vi "Decode Response.vi"(6 "error in (no error)":errorcluster, 9 "output cluster in":T1) -> (0 "error out":errorcluster, 3 "output cluster out":T1)   [LabVIEW 2020]
uses:
  Data Cluster.ctl
  <vilib>/Utility/miscctls.llb/LVDateTimeRec.ctl
panel:
  out "NumSamples":u8
  out "Samples (new, old, older)":u8[](array[numeric]) format="%02x"
  out "Status":u8
  out "Offset":u8
  out "Range":u8
  out "Sample (new)":sgl
  out "Sample (old)":sgl
  out "Sample (older)":sgl
  out "Mo":sgl
  out "unsigned byte array":u8[](array[numeric])
  out "Mf":sgl
  # "Send Data:"
  # "Receive Data:"
  # "Send Data:"
  # "Receive Data:"
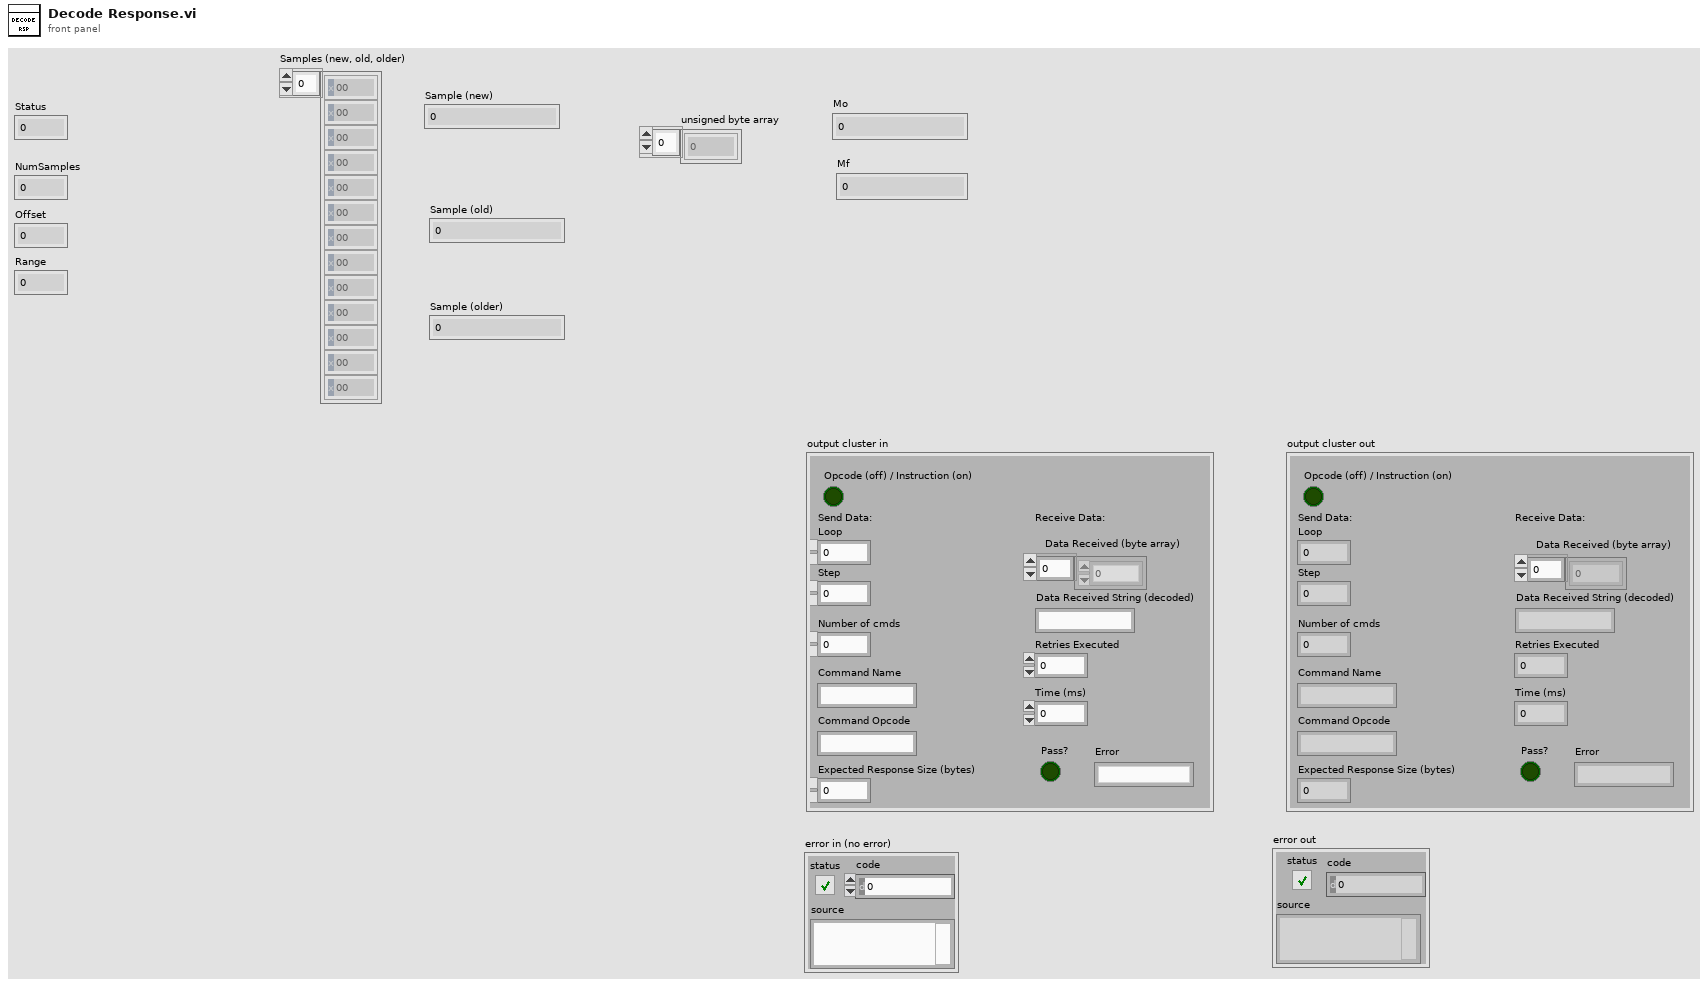
[diagram p1: front panel]
types:
  T1 = typedef "Data Cluster.ctl" = cluster{"Command Name":string, "Command Opcode ":string, "Step":dbl, "Loop":dbl, "Expected Response Size (bytes)":u16, "Number of cmds":dbl, "Data Received (byte array)":u8[], "Retries Executed":u16, "Time (ms)":u16, "Pass?":bool, "Opcode (off) / Instruction (on)":bool, "Data Received String (decoded)":string, "Error":string}
  T2 = typedef "LVDateTimeRec.ctl" = cluster{"fractional second":dbl, "second":i32, "minute":i32, "hour":i32, "day of month":i32, "month":i32, "year":i32, "day of week":i32, "day of year":i32, "DST":i32}
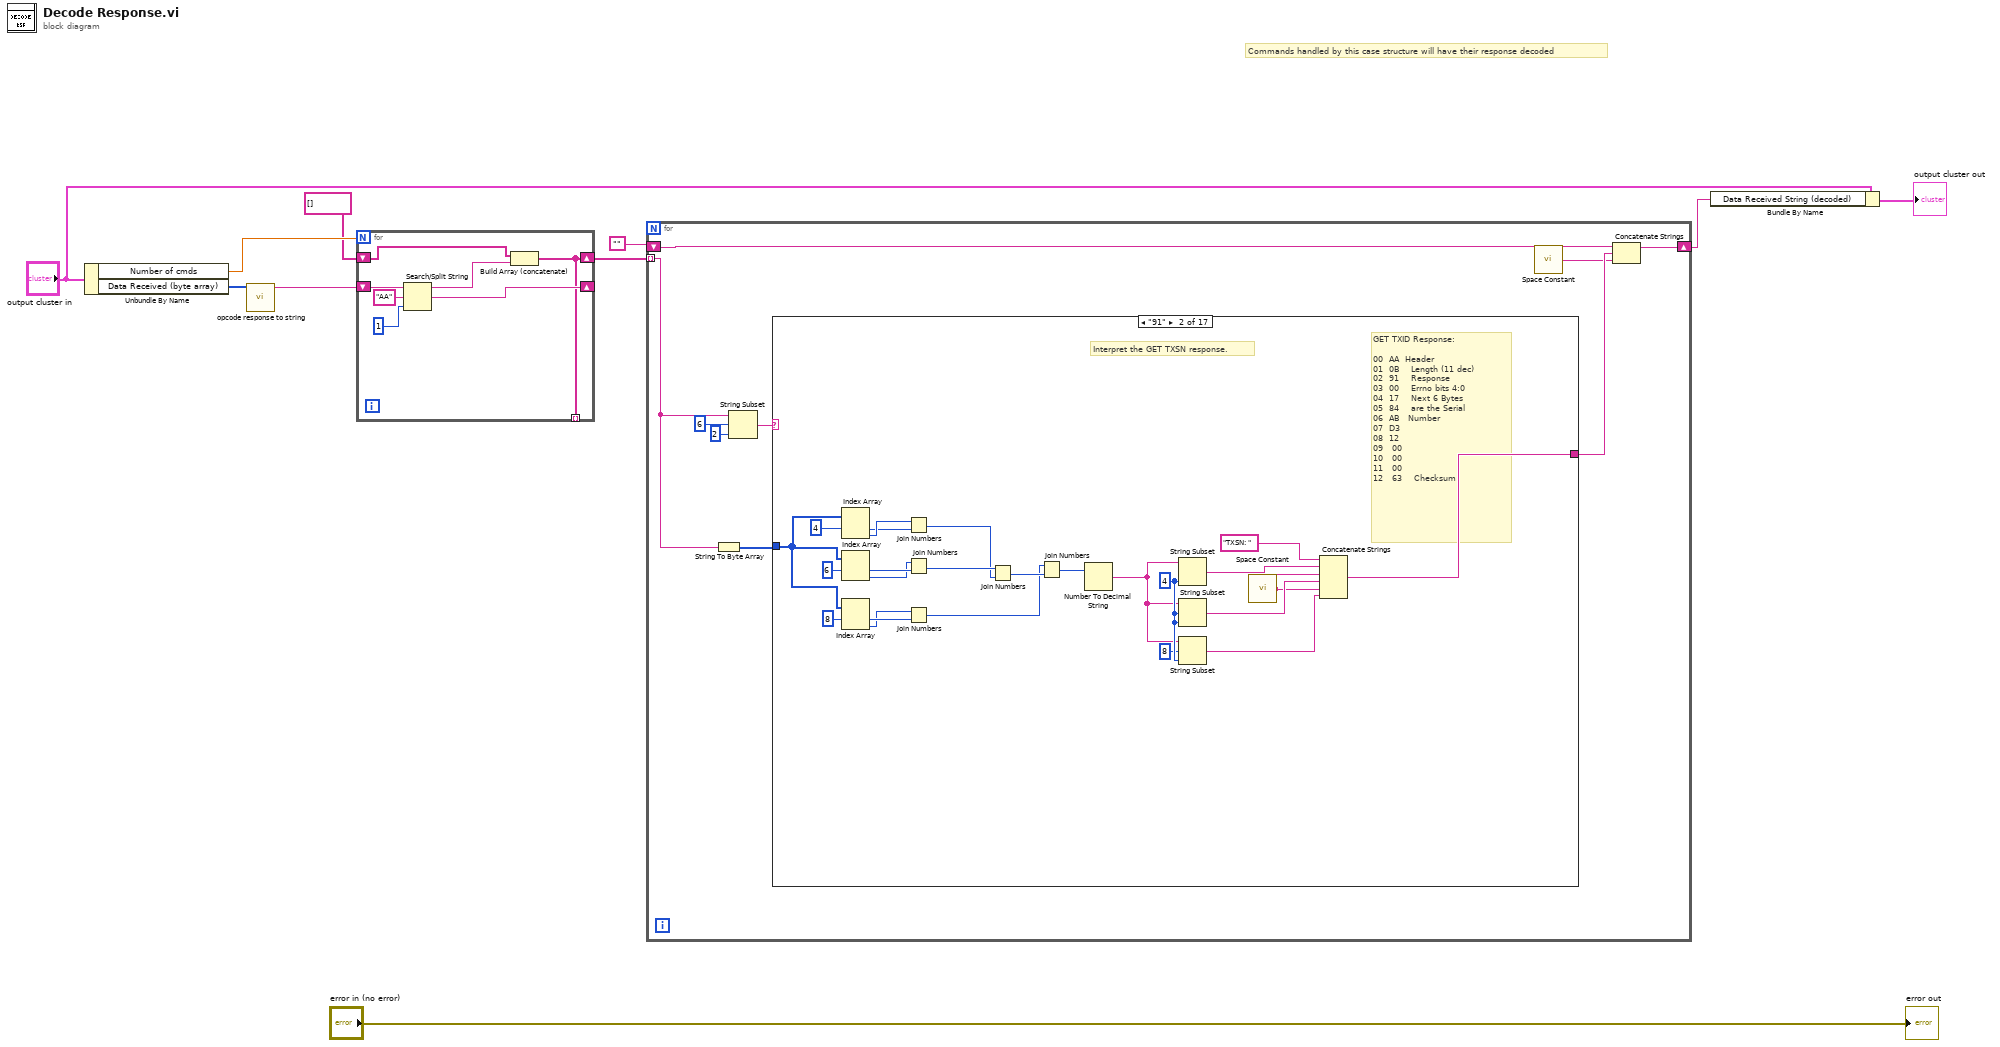
[diagram p0: block diagram]
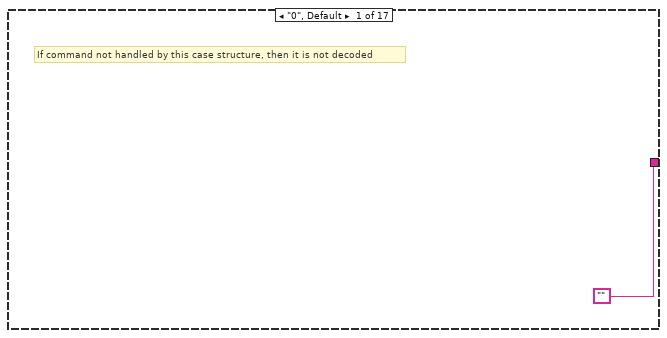
[diagram p2: hidden frame]
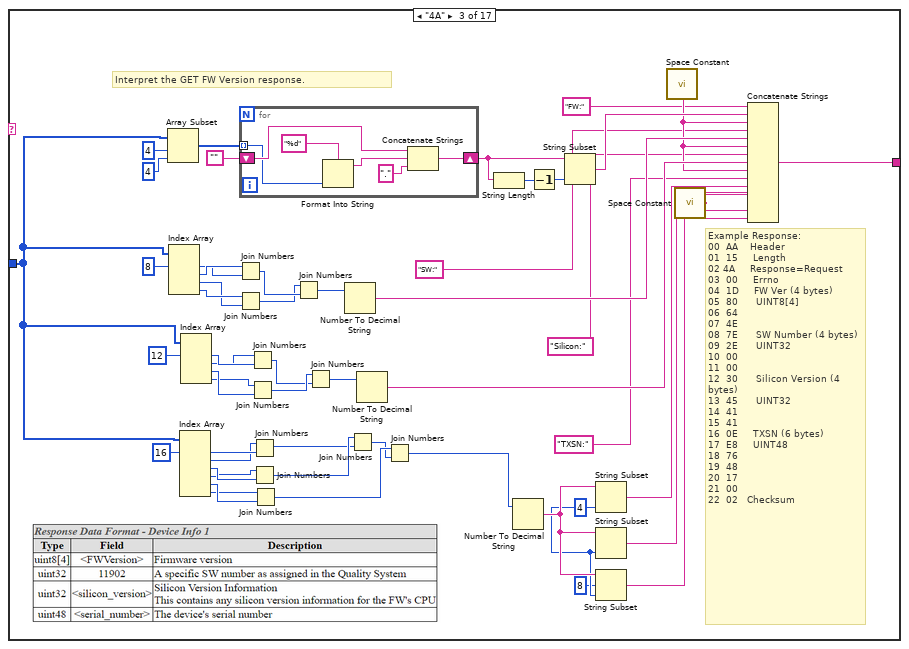
[diagram p3: hidden frame]
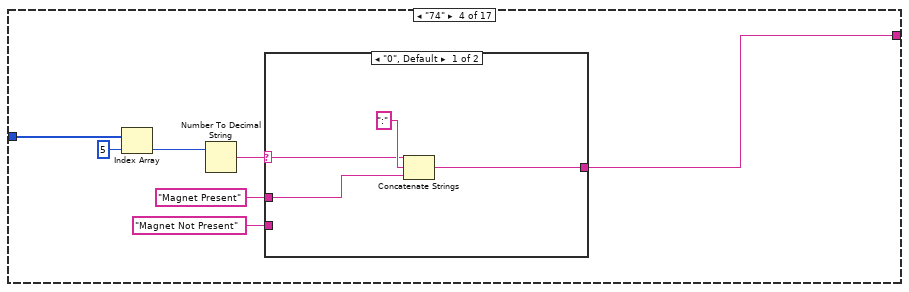
[diagram p4: hidden frame]
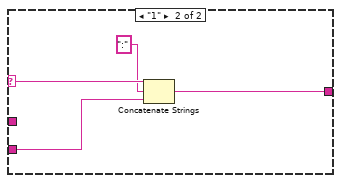
[diagram p5: hidden frame]
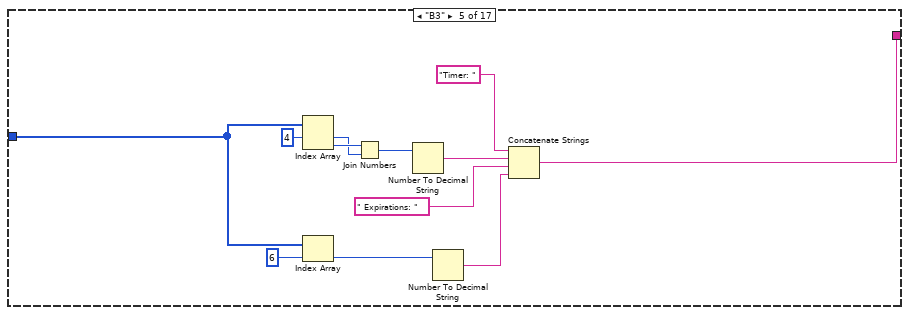
[diagram p6: hidden frame]
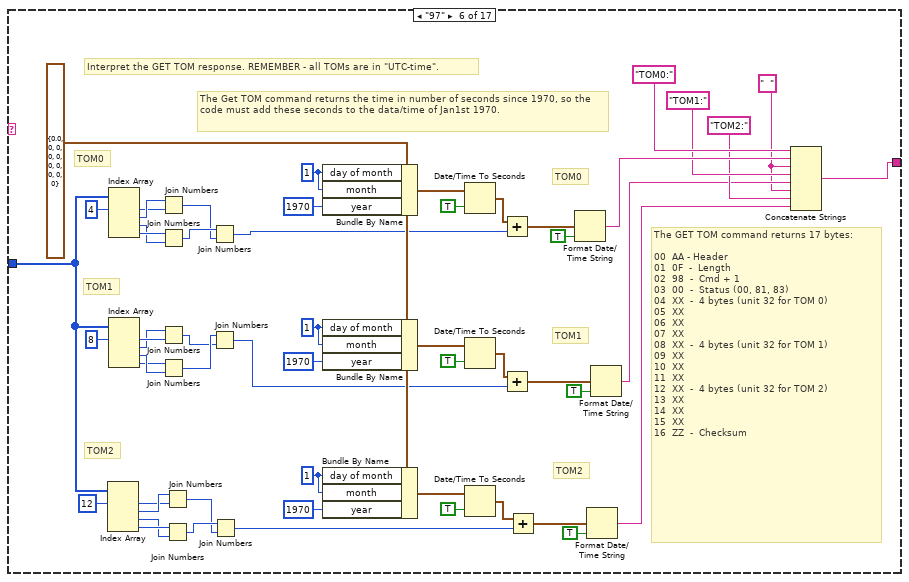
[diagram p7: hidden frame]
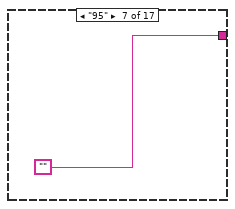
[diagram p8: hidden frame]
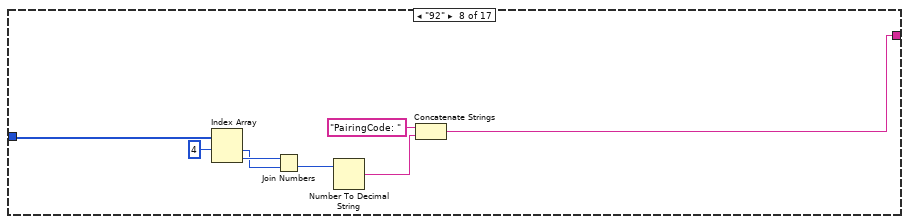
[diagram p9: hidden frame]
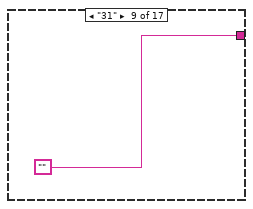
[diagram p10: hidden frame]
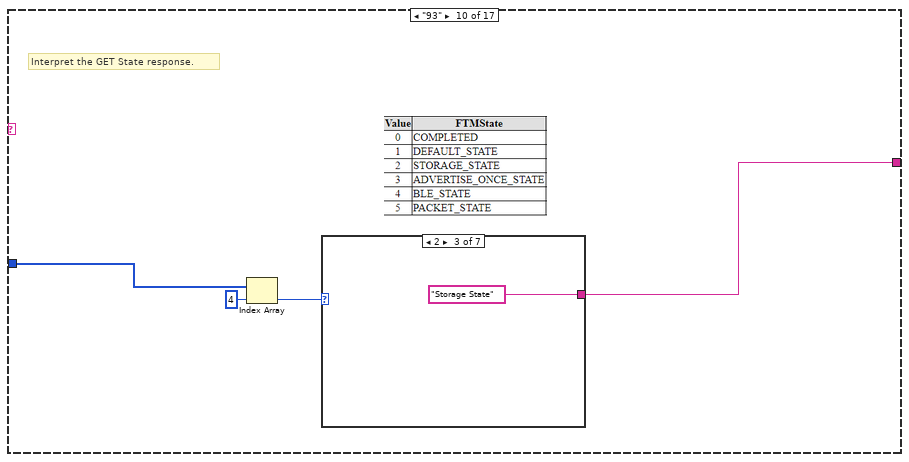
[diagram p11: hidden frame]
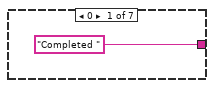
[diagram p12: hidden frame]
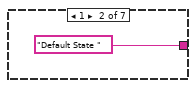
[diagram p13: hidden frame]
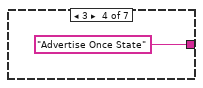
[diagram p14: hidden frame]
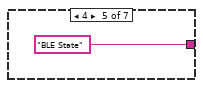
[diagram p15: hidden frame]
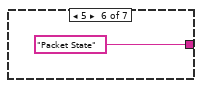
[diagram p16: hidden frame]
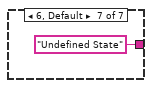
[diagram p17: hidden frame]
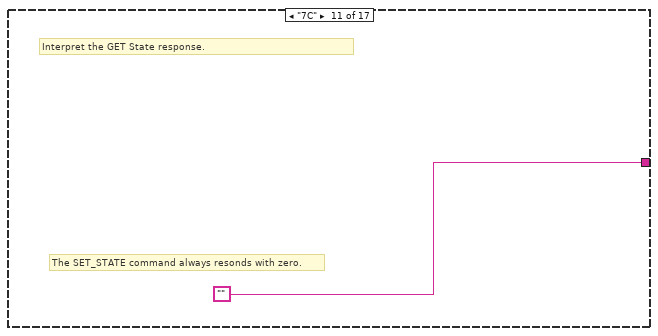
[diagram p18: hidden frame]
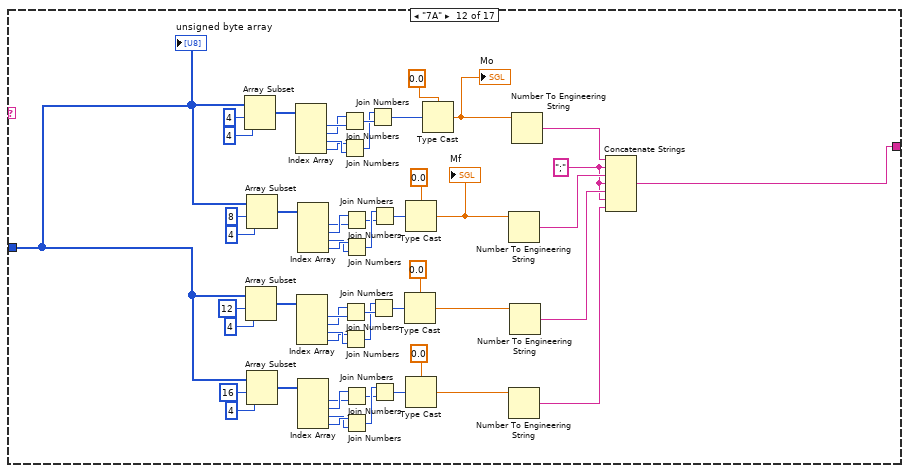
[diagram p19: hidden frame]
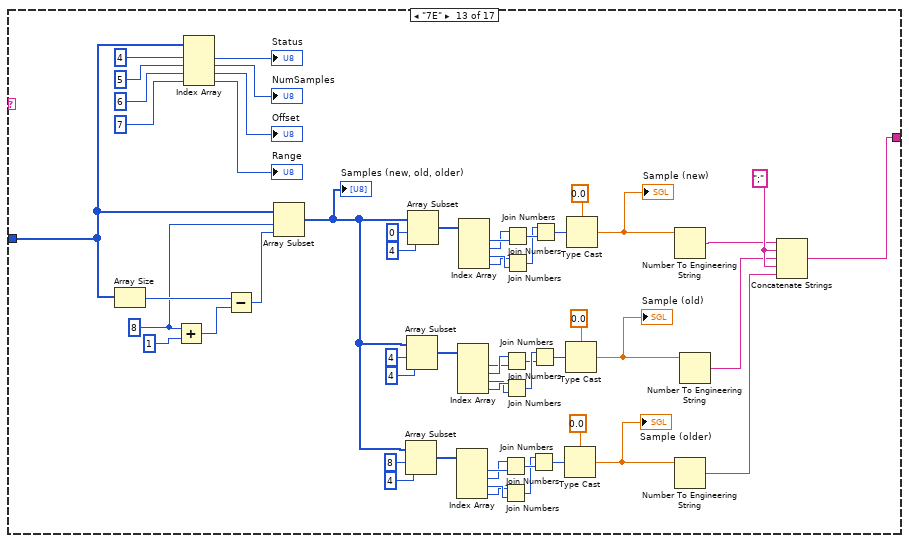
[diagram p20: hidden frame]
diagram:
  # "Commands handled by this case structure will have their response decoded"
  n1 = Unbundle By Name("output cluster in") -> ("Number of cmds"=w8:dbl, "Data Received (byte array)"=w7:u8[])
  n2 = call "opcode response to string.vi"("Data Received"=w7) -> ("Response String"=w6:string)  [unwired: 10 in]
  n3 = for {
    N: w8 -> [_]
    shift-right: [w11] -> w4
    shift-left: string[] [] -> [w13]
    shift-right: [w12] -> _
    shift-left: w6 -> [w16]
    tunnel: [w11] -> _ mode=indexing
    n4 = Search/Split String(string=w16, search string/char (-)="AA", offset (0)=1) -> (substring before match=w14:string, match + rest of string=w12:string)  [unwired: 1 out]
    n5 = Build Array (concatenate)(w13, w14) -> (w11:string[])
  }
  n6 = for {
    tunnel: w4 -> [w21] mode=indexing
    shift-right: [w26] -> w3
    shift-left: "" -> [w25]
    n7 = String To Byte Array(string=w21) -> (unsigned byte array=w24:u8[])
    n8 = String Subset(string=w21, offset (0)=6, length (rest)=2 ("length (rest)")) -> (substring=w23:string)
    n9 = case shown="\"91\"" w23 {
      tunnel: w24 -> [_ w45 w67 w115 w126 w144 _ w197 _ w203 _ w219 w270 w329 w349 w361 _]
      tunnel: ["" w41 w66 w110 w127 w143 "" w193 "" w202 "" w242 w269 w328 w340 w359 ""] -> w19
      frame "0", Default {
        # "If command not handled by this case structure, then it is not decoded"
      }
      frame "91" {
        w34 = 4 ("length (rest)")
        # "GET TXID Response:\n\n00  AA  Header\n01  0B    Length (11 dec)\n02  91    Response\n03  00    Errno bits 4:0\n04  17    Next 6 Bytes \n05  84    are the Serial\n06  AB   Number\n07  D3\n08  12\n09   00\n10   00\n11   00\n12   63    Checksum"
        # "Interpret the GET TXSN response."
        n10 = Index Array(array=w45, index #1=6 ("index")) -> (element #1=w43:u8, element #2=w42:u8)  [unwired: 1 in]
        n11 = Index Array(array=w45, index #1=4 ("index")) -> (element #1=w49:u8, element #2=w50:u8)  [unwired: 1 in]
        n12 = Index Array(array=w45, index #1=8 ("index")) -> (element #1=w46:u8, element #2=w44:u8)  [unwired: 1 in]
        n13 = Join Numbers(hi=w50, lo=w49) -> ((hi.lo)=w38:u16)
        n14 = Join Numbers(hi=w42, lo=w43) -> ((hi.lo)=w39:u16)
        n15 = Join Numbers(hi=w44, lo=w46) -> ((hi.lo)=w36:u16)
        n16 = Join Numbers(hi=w39, lo=w38) -> ((hi.lo)=w37:u32)
        n17 = Join Numbers(hi=w36, lo=w37) -> ((hi.lo)=w35:u64)
        n18 = Number To Decimal String(number=w35) -> (decimal integer string=w32:string)  [unwired: 1 in]
        n19 = String Subset(string=w32, length (rest)=w34) -> (substring=w31:string)  [unwired: 1 in]
        n20 = String Subset(string=w32, offset (0)=w34, length (rest)=w34) -> (substring=w30:string)
        n21 = String Subset(string=w32, offset (0)=8, length (rest)=w34) -> (substring=w28:string)
        n22 = call <vilib>:"Space Constant.vi"() -> ("String"=w29:string)
        n23 = Concatenate Strings("TXSN: " ("String"), w31, w29, w30, w29, w28) -> (w41:string)
      }
      frame "4A" {
        w79 = 4 ("length (rest)")
        # "Example Response:\n00  AA    Header\n01  15     Length\n02 4A     Response=Request\n03  00     Errno\n04  1D     FW Ver (4 bytes)   \n05  80      UINT8[4]\n06  64    \n07  4E    \n08  7E      SW Number (4 bytes)\n09  2E      UINT32\n10  00\n11  00\n12  30      Silicon Version (4 bytes)\n13  45      UINT32\n14  41\n15  41     \n16  0E     TXSN (6 bytes)\n17  E8     UINT48\n18  76    \n19  48\n20  17\n21  00\n22  02   Checksum"
        # "Interpret the GET FW Version response."
        n24 = Array Subset(array=w67, index=4, length=4) -> (w85:u8[])
        n25 = Index Array(array=w67, index #1=8 ("index")) -> (element #1=w64:u8, element #2=w65:u8, element #3=w62:u8, element #4=w63:u8)  [unwired: 3 in]
        n26 = Index Array(array=w67, index #1=16 ("index")) -> (element #1=w57:u8, element #2=w56:u8, element #3=w55:u8, element #4=w54:u8, element #5=w53:u8, element #6=w52:u8)  [unwired: 5 in]
        n27 = Index Array(array=w67, index #1=12 ("index")) -> (element #1=w61:u8, element #2=w60:u8, element #3=w59:u8, element #4=w58:u8)  [unwired: 3 in]
        n28 = Join Numbers(hi=w65, lo=w64) -> ((hi.lo)=w87:u16)
        n29 = Join Numbers(hi=w63, lo=w62) -> ((hi.lo)=w86:u16)
        n30 = for {
          tunnel: w85 -> [w104] mode=indexing
          shift-right: [w106] -> w84
          shift-left: "" -> [w108]
          n31 = Format Into String(format string="%d", w104) -> (resulting string=w107:string)  [unwired: 2 in, 1 out]
          n32 = Concatenate Strings(w108, w107, "." ("string")) -> (w106:string)
        }
        n33 = Join Numbers(hi=w60, lo=w61) -> ((hi.lo)=w91:u16)
        n34 = Join Numbers(hi=w58, lo=w59) -> ((hi.lo)=w92:u16)
        n35 = Join Numbers(hi=w56, lo=w57) -> ((hi.lo)=w99:u16)
        n36 = Join Numbers(hi=w54, lo=w55) -> ((hi.lo)=w100:u16)
        n37 = Join Numbers(hi=w52, lo=w53) -> ((hi.lo)=w102:u16)
        n38 = Join Numbers(hi=w86, lo=w87) -> ((hi.lo)=w88:u32)
        n39 = Join Numbers(hi=w92, lo=w91) -> ((hi.lo)=w90:u32)
        n40 = Number To Decimal String(number=w88) -> (decimal integer string=w89:string)  [unwired: 1 in]
        n41 = Join Numbers(hi=w100, lo=w99) -> ((hi.lo)=w101:u32)
        n42 = Number To Decimal String(number=w90) -> (decimal integer string=w93:string)  [unwired: 1 in]
        n43 = Join Numbers(hi=w102, lo=w101) -> ((hi.lo)=w103:u64)
        n44 = String Length(string=w84) -> (length=w83:i32)
        n45 = Number To Decimal String(number=w103) -> (decimal integer string=w98:string)  [unwired: 1 in]
        n46 = Decrement(x=w83) -> (x-1=w82:i32)
        n47 = String Subset(string=w84, length (rest)=w82) -> (substring=w81:string)  [unwired: 1 in]
        n48 = String Subset(string=w98, length (rest)=w79) -> (substring=w95:string)  [unwired: 1 in]
        n49 = String Subset(string=w98, offset (0)=w79, length (rest)=w79) -> (substring=w96:string)
        n50 = String Subset(string=w98, offset (0)=8, length (rest)=w79) -> (substring=w97:string)
        n51 = call <vilib>:"Space Constant.vi"() -> ("String"=w80:string)
        n52 = call <vilib>:"Space Constant.vi"() -> ("String"=w94:string)
        n53 = Concatenate Strings("FW:", w81, w80, "SW:", w89, w80, "Silicon:", w93, w80, "TXSN:", w95, w94, w96, w94, w97) -> (w66:string)
      }
      frame "74" {
        n54 = Index Array(array=w115, index=5) -> (element=w114:u8)
        n55 = Number To Decimal String(number=w114) -> (decimal integer string=w113:string)  [unwired: 1 in]
        n56 = case shown="\"0\", Default" w113 {
          selector: w113 -> [w119 w124]
          tunnel: "Magnet Not Present" -> [_ w122]
          tunnel: "Magnet Present" -> [w118 _]
          tunnel: [w117 w121] -> w110
          frame "0", Default {
            n57 = Concatenate Strings(w119, ":", w118) -> (w117:string)
          }
          frame "1" {
            n58 = Concatenate Strings(w124, ":", w122) -> (w121:string)
          }
        }
      }
      frame "B3" {
        n59 = Index Array(array=w126, index #1=4 ("index")) -> (element #1=w134:u8, element #2=w135:u8)  [unwired: 1 in]
        n60 = Index Array(array=w126, index=6) -> (element=w133:u8)
        n61 = Join Numbers(hi=w135, lo=w134) -> ((hi.lo)=w136:u16)
        n62 = Number To Decimal String(number=w136) -> (decimal integer string=w129:string)  [unwired: 1 in]
        n63 = Number To Decimal String(number=w133) -> (decimal integer string=w128:string)  [unwired: 1 in]
        n64 = Concatenate Strings("Timer: " ("string"), w129, " Expirations: " ("string"), w128) -> (w127:string)
      }
      frame "97" {
        w137 = "  "
        w159 = 1 ("day of month")
        w162 = 1 ("day of month")
        w169 = 1 ("day of month")
        w155 = T2 {"fractional second"=0.0, "second"=0, "minute"=0, "hour"=0, "day of month"=0, "month"=0, "year"=0, "day of week"=0, "day of year"=0, "DST"=0} ("date time rec")
        # "TOM2"
        # "TOM1"
        # "TOM0"
        # "TOM2"
        # "TOM1"
        # "TOM0"
        # "Interpret the GET TOM response. REMEMBER - all TOMs are in \"UTC-time\"."
        # "The GET TOM command returns 17 bytes:\n\n00  AA - Header\n01  0F  -  Length\n02  98  -  Cmd + 1\n03  00  -  Status (00, 81, 83)\n04  XX  -  4 bytes (unit 32 for TOM 0)\n05  XX\n06  XX\n07  XX\n08  XX  -  4 bytes (unit 32 for TOM 1)\n09  XX\n10  XX\n11  XX\n12  XX  -  4 bytes (unit 32 for TOM 2)\n13  XX\n14  XX\n15  XX\n16  ZZ  -  Checksum"
        # "The Get TOM command returns the time in number of seconds since 1970, so the code must add these seconds to the data/time of Jan1st 1970."
        n65 = Index Array(array=w144, index #1=12 ("index")) -> (element #1=w179:u8, element #2=w180:u8, element #3=w177:u8, element #4=w178:u8)  [unwired: 3 in]
        n66 = Index Array(array=w144, index #1=4 ("index")) -> (element #1=w189:u8, element #2=w190:u8, element #3=w187:u8, element #4=w188:u8)  [unwired: 3 in]
        n67 = Index Array(array=w144, index #1=8 ("index")) -> (element #1=w184:u8, element #2=w183:u8, element #3=w186:u8, element #4=w185:u8)  [unwired: 3 in]
        n68 = Join Numbers(hi=w190, lo=w189) -> ((hi.lo)=w175:u16)
        n69 = Join Numbers(hi=w188, lo=w187) -> ((hi.lo)=w176:u16)
        n70 = Join Numbers(hi=w183, lo=w184) -> ((hi.lo)=w173:u16)
        n71 = Join Numbers(hi=w185, lo=w186) -> ((hi.lo)=w174:u16)
        n72 = Join Numbers(hi=w180, lo=w179) -> ((hi.lo)=w171:u16)
        n73 = Join Numbers(hi=w178, lo=w177) -> ((hi.lo)=w172:u16)
        n74 = Join Numbers(hi=w176, lo=w175) -> ((hi.lo)=w154:u32)
        n75 = Join Numbers(hi=w174, lo=w173) -> ((hi.lo)=w153:u32)
        n76 = Join Numbers(hi=w172, lo=w171) -> ((hi.lo)=w152:u32)
        n77 = Bundle By Name(cluster=w155, "day of month"=w169, "month"=w169, "year"=1970) -> (w170:T2)
        n78 = Bundle By Name(cluster=w155, "day of month"=w162, "month"=w162, "year"=1970) -> (w161:T2)
        n79 = Bundle By Name(cluster=w155, "day of month"=w159, "month"=w159, "year"=1970) -> (w160:T2)
        n80 = Date/Time To Seconds(1:TRUE ("is UTC (F)"), 2:w170) -> (0:w166:timestamp)
        n81 = Date/Time To Seconds(1:TRUE ("is UTC (F)"), 2:w161) -> (0:w165:timestamp)
        n82 = Date/Time To Seconds(1:TRUE ("is UTC (F)"), 2:w160) -> (0:w156:timestamp)
        n83 = Add(x=w166, y=w154) -> (x+y=w146:timestamp)
        n84 = Add(x=w165, y=w153) -> (x+y=w147:timestamp)
        n85 = Add(x=w156, y=w152) -> (x+y=w151:timestamp)
        n86 = Format Date/Time String(seconds (now)=w146, UTC format=TRUE) -> (date/time string=w145:string)  [unwired: 1 in]
        n87 = Format Date/Time String(seconds (now)=w151, UTC format=TRUE) -> (date/time string=w140:string)  [unwired: 1 in]
        n88 = Format Date/Time String(seconds (now)=w147, UTC format=TRUE) -> (date/time string=w138:string)  [unwired: 1 in]
        n89 = Concatenate Strings("TOM0:", w145, w137, "TOM1:", w138, w137, "TOM2:", w140) -> (w143:string)
      }
      frame "95" {
      }
      frame "92" {
        n90 = Index Array(array=w197, index #1=4 ("index")) -> (element #1=w199:u8, element #2=w200:u8)  [unwired: 1 in]
        n91 = Join Numbers(hi=w200, lo=w199) -> ((hi.lo)=w196:u16)
        n92 = Number To Decimal String(number=w196) -> (decimal integer string=w195:string)  [unwired: 1 in]
        n93 = Concatenate Strings("PairingCode: " ("string"), w195) -> (w193:string)
      }
      frame "31" {
      }
      frame "93" {
        # "Interpret the GET State response."
        n94 = Index Array(array=w203, index=4) -> (element=w204:u8)
        n95 = case shown="2" w204 {
          tunnel: ["Completed " "Default State " "Storage State" "Advertise Once State" "BLE State" "Packet State" "Undefined State"] -> w202
          frame 0 {
          }
          frame 1 {
          }
          frame 2 {
          }
          frame 3 {
          }
          frame 4 {
          }
          frame 5 {
          }
          frame 6, Default {
          }
        }
      }
      frame "7C" {
        # "The SET_STATE command always resonds with zero."
        # "Interpret the GET State response."
      }
      frame "7A" {
        w215 = ";"
        n96 = Array Subset(array=w219, index=4, length=4) -> (w258:u8[])
        n97 = Array Subset(array=w219, index=12, length=4) -> (w231:u8[])
        n98 = Array Subset(array=w219, index=8, length=4) -> (w256:u8[])
        n99 = Array Subset(array=w219, index=16, length=4) -> (w230:u8[])
        n100 = Index Array(array=w258) -> (element #1=w266:u8, element #2=w265:u8, element #3=w264:u8, element #4=w263:u8)  [unwired: 4 in]
        n101 = Index Array(array=w231) -> (element #1=w239:u8, element #2=w238:u8, element #3=w237:u8, element #4=w236:u8)  [unwired: 4 in]
        n102 = Index Array(array=w256) -> (element #1=w248:u8, element #2=w249:u8, element #3=w250:u8, element #4=w251:u8)  [unwired: 4 in]
        n103 = Index Array(array=w230) -> (element #1=w222:u8, element #2=w223:u8, element #3=w224:u8, element #4=w225:u8)  [unwired: 4 in]
        n104 = Join Numbers(hi=w265, lo=w266) -> ((hi.lo)=w262:u16)
        n105 = Join Numbers(hi=w263, lo=w264) -> ((hi.lo)=w261:u16)
        n106 = Join Numbers(hi=w238, lo=w239) -> ((hi.lo)=w235:u16)
        n107 = Join Numbers(hi=w236, lo=w237) -> ((hi.lo)=w234:u16)
        n108 = Join Numbers(hi=w249, lo=w248) -> ((hi.lo)=w252:u16)
        n109 = Join Numbers(hi=w251, lo=w250) -> ((hi.lo)=w253:u16)
        n110 = Join Numbers(hi=w223, lo=w222) -> ((hi.lo)=w226:u16)
        n111 = Join Numbers(hi=w225, lo=w224) -> ((hi.lo)=w227:u16)
        n112 = Join Numbers(hi=w261, lo=w262) -> ((hi.lo)=w260:u32)
        n113 = Join Numbers(hi=w234, lo=w235) -> ((hi.lo)=w233:u32)
        n114 = Join Numbers(hi=w253, lo=w252) -> ((hi.lo)=w254:u32)
        n115 = Join Numbers(hi=w227, lo=w226) -> ((hi.lo)=w228:u32)
        n116 = Type Cast(type=sgl 0.0, x=w233) -> (*(type *) &x=w218:sgl)
        n117 = Type Cast(type=sgl 0.0, x=w254) -> (*(type *) &x=w245:sgl)
        "Mf" <- w245
        n118 = Type Cast(type=sgl 0.0, x=w228) -> (*(type *) &x=w217:sgl)
        n119 = Type Cast(type=sgl 0.0, x=w260) -> (*(type *) &x=w257:sgl)
        "Mo" <- w257
        n120 = Number To Engineering String(4:w245) -> (0:w243:string)  [unwired: 3 in]
        n121 = Number To Engineering String(4:w217) -> (0:w214:string)  [unwired: 3 in]
        n122 = Number To Engineering String(4:w218) -> (0:w216:string)  [unwired: 3 in]
        n123 = Number To Engineering String(4:w257) -> (0:w244:string)  [unwired: 3 in]
        n124 = Concatenate Strings(w244, w215, w243, w215, w216, w215, w214) -> (w242:string)
        "unsigned byte array" <- w219
      }
      frame "7E" {
        w274 = ";"
        w322 = 8 ("index")
        n125 = Array Size(array=w270) -> (size(s)=w323:i32)
        n126 = Add(x=w322, y=1) -> (x+y=w320:i32)
        n127 = Index Array(array=w270, index #1=4 ("index"), index #2=5 ("index"), index #3=6 ("index"), index #4=7 ("index")) -> (element #1=→"Status":u8, element #2=→"NumSamples":u8, element #3=→"Offset":u8, element #4=→"Range":u8)
        n128 = Subtract(x=w323, y=w320) -> (x-y=w319:i32)
        n129 = Array Subset(array=w270, index=w322, length=w319) -> (w280:u8[])
        "Samples (new, old, older)" <- w280
        n130 = Array Subset(array=w280, index=8, length=4) -> (w281:u8[])
        n131 = Array Subset(array=w280, index=4, length=4) -> (w302:u8[])
        n132 = Array Subset(array=w280, index=0, length=4) -> (w303:u8[])
        n133 = Index Array(array=w281) -> (element #1=w289:u8, element #2=w288:u8, element #3=w287:u8, element #4=w286:u8)  [unwired: 4 in]
        n134 = Index Array(array=w302) -> (element #1=w294:u8, element #2=w295:u8, element #3=w296:u8, element #4=w297:u8)  [unwired: 4 in]
        n135 = Index Array(array=w303) -> (element #1=w311:u8, element #2=w310:u8, element #3=w309:u8, element #4=w308:u8)  [unwired: 4 in]
        n136 = Join Numbers(hi=w288, lo=w289) -> ((hi.lo)=w285:u16)
        n137 = Join Numbers(hi=w286, lo=w287) -> ((hi.lo)=w284:u16)
        n138 = Join Numbers(hi=w295, lo=w294) -> ((hi.lo)=w298:u16)
        n139 = Join Numbers(hi=w297, lo=w296) -> ((hi.lo)=w299:u16)
        n140 = Join Numbers(hi=w310, lo=w311) -> ((hi.lo)=w307:u16)
        n141 = Join Numbers(hi=w308, lo=w309) -> ((hi.lo)=w306:u16)
        n142 = Join Numbers(hi=w284, lo=w285) -> ((hi.lo)=w283:u32)
        n143 = Join Numbers(hi=w299, lo=w298) -> ((hi.lo)=w300:u32)
        n144 = Join Numbers(hi=w306, lo=w307) -> ((hi.lo)=w305:u32)
        n145 = Type Cast(type=sgl 0.0, x=w283) -> (*(type *) &x=w275:sgl)
        "Sample (older)" <- w275
        n146 = Type Cast(type=sgl 0.0, x=w300) -> (*(type *) &x=w276:sgl)
        "Sample (old)" <- w276
        n147 = Type Cast(type=sgl 0.0, x=w305) -> (*(type *) &x=w277:sgl)
        "Sample (new)" <- w277
        n148 = Number To Engineering String(4:w277) -> (0:w273:string)  [unwired: 3 in]
        n149 = Number To Engineering String(4:w275) -> (0:w271:string)  [unwired: 3 in]
        n150 = Number To Engineering String(4:w276) -> (0:w272:string)  [unwired: 3 in]
        n151 = Concatenate Strings(w273, w274, w272, w274, w271) -> (w269:string)
      }
      frame "22" {
        # "Interpret the GET Battery Voltages response."
        # "Voltages: Satatic, Dynamic"
        n152 = Index Array(array=w329, index #1=4 ("index")) -> (element #1=w337:u8, element #2=w336:u8)  [unwired: 1 in]
        n153 = Index Array(array=w329, index #1=6 ("index")) -> (element #1=w339:u8, element #2=w338:u8)  [unwired: 1 in]
        n154 = Join Numbers(hi=w336, lo=w337) -> ((hi.lo)=w333:u16)
        n155 = Join Numbers(hi=w338, lo=w339) -> ((hi.lo)=w332:u16)
        n156 = Number To Decimal String(number=w333) -> (decimal integer string=w331:string)  [unwired: 1 in]
        n157 = Number To Decimal String(number=w332) -> (decimal integer string=w326:string)  [unwired: 1 in]
        n158 = Concatenate Strings("Static:" ("string"), w331, "  ", "Dynamic:" ("string"), w326) -> (w328:string)
      }
      frame "C2" {
        # "Interpret the GET Temperature response."
        # "This is a bitmask of enabled and detected temperature sensors."
        # "Get Temp Response Format:\n\nAA  -  Header\n08    -  Length \nC3   -  Response (C2+1)\n00   -  Tx Status\n57    -  Bit-masked Temp Status (57 desired)\nD0   -  centi-degrees C (4 bytes) unit 32\n08\n00\n00 \n44   -  Checksum"
        # "Temp"
        # "Status (should be 0x57)"
        n159 = Index Array(array=w349, index #1=4 ("index")) -> (element #1=w346:u8, element #2=w348:u8, element #3=w355:u8)  [unwired: 2 in]
        n160 = Join Numbers(hi=w355, lo=w348) -> ((hi.lo)=w353:u16)
        n161 = Divide(x=w353, y=u16 100) -> (x/y=w351:dbl)
        n162 = Format Into String(format string="%02x", w346) -> (resulting string=w342:string)  [unwired: 2 in, 1 out]
        n163 = Number To Fractional String(number=w351, precision (6)=i16 2) -> (F-format string=w345:string)  [unwired: 2 in]
        n164 = Concatenate Strings("Temp:" ("string"), w345, "   ", "Status:" ("string"), w342) -> (w340:string)
      }
      frame "56" {
        # "Interpret the GET Battery Type response."
        n165 = Index Array(array=w361, index=6) -> (element=w358:u8)
        n166 = Number To Decimal String(number=w358) -> (decimal integer string=w357:string)  [unwired: 1 in]
        n167 = case shown="\"0\", Default" w357 {
          tunnel: ["Panasonic" "Murata" "Invalid" "Invalid" "Maxell" "Invalid" "Invalid"] -> w356
          frame "5" {
          }
          frame "6" {
          }
          frame "0", Default {
          }
          frame "1" {
          }
          frame "2" {
          }
          frame "3" {
          }
          frame "4" {
          }
        }
        n168 = Concatenate Strings("Type:", w356) -> (w359:string)
      }
      frame "4D" {
        # "The SET_STATE command has no response text."
        # "0x4E: Convert the Switch from CGM to FTM Mode (0x4D) Response"
      }
    }
    n169 = call <vilib>:"Space Constant.vi"() -> ("String"=w18:string)
    n170 = Concatenate Strings(w25, w19, w18) -> (w26:string)
  }
  n171 = Bundle By Name(cluster="output cluster in", "Data Received String (decoded)"=w3) -> (→"output cluster out":T1)
  "error out" <- "error in (no error)"
